vi "playwright-testing-event.vi"() -> ()   [LabVIEW 2023]
panel:
  out "register array":T1(array[cluster])
  out "available event":T1(array[cluster])
  out "Init event":T1(array[cluster])
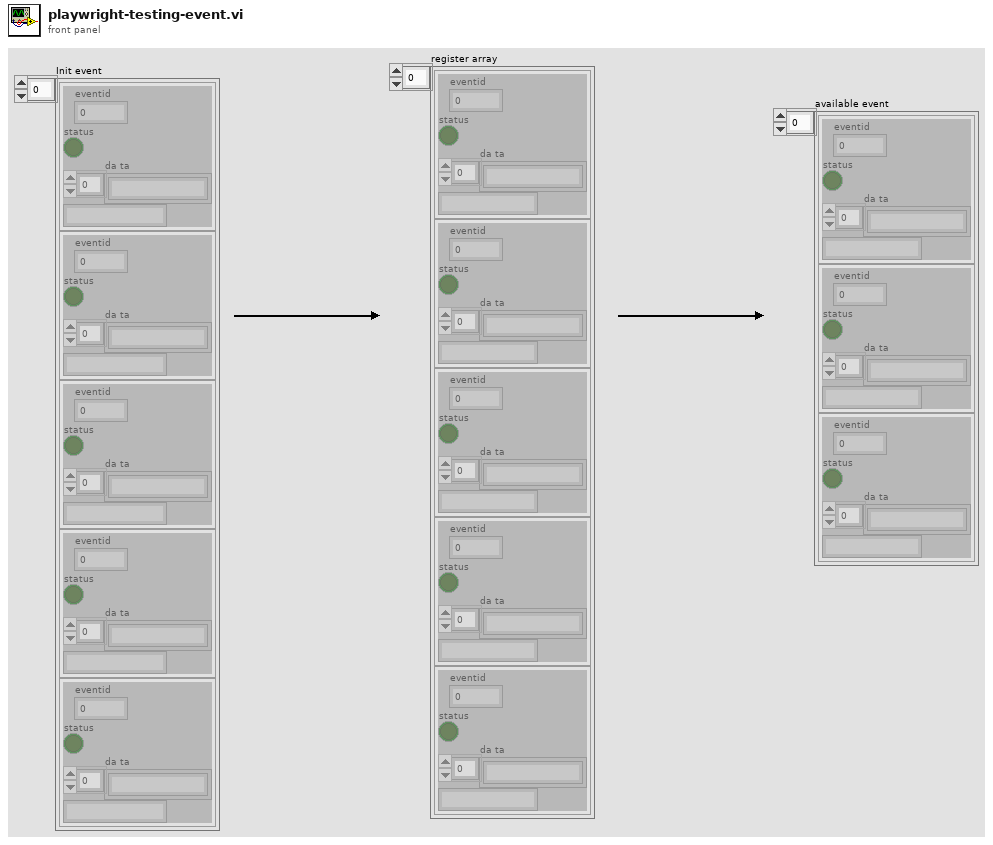
[diagram p1: front panel]
types:
  T1 = cluster{"eventid":dbl, "status":bool, "da ta":string[], string}[]
  T2 = cluster{"eventid":dbl, "status":bool, "da ta":string[], string}
  T3 = cluster{"eventid":dbl, bool, "da ta":string[], string}
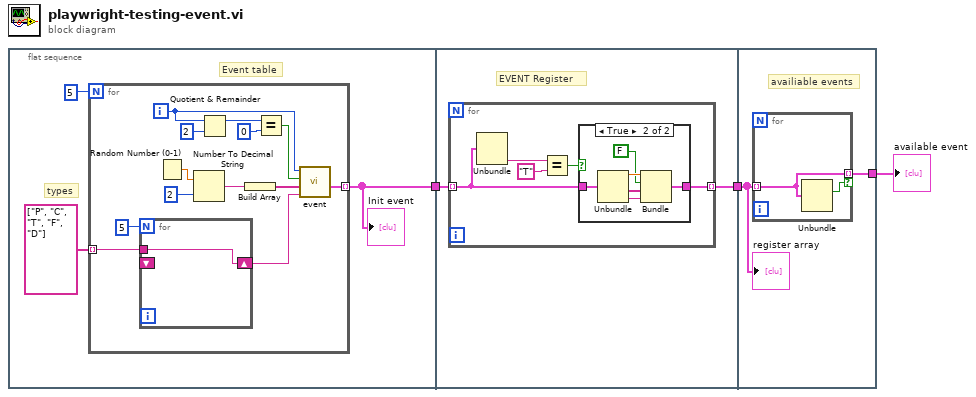
[diagram p0: block diagram]
diagram:
  n1 = flat-sequence {
    tunnel: [w5] -> w3
    tunnel: w3 -> [w22]
    tunnel: [w21] -> w2
    tunnel: w2 -> [w35]
    tunnel: [w36] -> w1
    frame #0 {
      # "types"
      # "Event table"
      n2 = for {
        N: 5 -> [_]
        tunnel: [w9] -> w5 mode=indexing
        tunnel: string[] ["P", "C", "T", "F", "D"] -> [w8] mode=indexing
        i -> [w16]
        n3 = for {
          N: 5 -> [_]
          shift-right: [w20] -> w10
          shift-left: _ -> [_]
          tunnel: w8 -> [w20]
        }
        n4 = Random Number (0-1)() -> (number: 0 to 1=w13:dbl)
        n5 = Number To Decimal String(number=w13, width (-)=i16 2) -> (decimal integer string=w12:string)
        n6 = Quotient & Remainder(x=w16, y=2) -> (x-y*floor(x/y)=w18:i32)  [unwired: 1 out]
        n7 = Build Array(w12) -> (w11:string[])
        n8 = Equal?(x=w18, y=0) -> (x = y?=w15:bool)
        n9 = call "event.vi"("type"=w10, "da ta"=w11, "status"=w15, "eventid"=w16) -> ("output cluster"=w9:T2)  [unwired: 7 in]
      }
      "Init event" <- w5
    }
    frame #1 {
      # "EVENT Register"
      n10 = for {
        tunnel: w22 -> [w25] mode=indexing
        tunnel: [w23] -> w21 mode=indexing
        n11 = Unbundle(w25) -> (w27:string)  [unwired: 3 out]
        n12 = Equal?(x=w27, y="T") -> (x = y?=w24:bool)
        n13 = case shown="True" w24 {
          tunnel: w25 -> [w28 w34]
          tunnel: [w28 w29] -> w23
          frame False {
          }
          frame True {
            n14 = Unbundle(w34) -> ("eventid"=w33:dbl, "da ta"=w31:string[], w30:string)  [unwired: 1 out]
            n15 = Bundle("eventid"=w33, FALSE, "da ta"=w31, w30) -> (w29:T3)  [unwired: 1 in]
          }
        }
      }
    }
    frame #2 {
      # "availiable events"
      n16 = for {
        tunnel: w35 -> [w38] mode=indexing
        tunnel: [w38] -> w36 mode=indexing if=w37
        n17 = Unbundle(w38) -> ("status"=w37:bool)  [unwired: 3 out]
      }
      "register array" <- w35
    }
  }
  "available event" <- w1
